vi "Drive Controller.vi"(8 "error in":errorcluster) -> ()   [LabVIEW 2015]
doc: "This VI executes continuously carrying out the current operation and responding to updates or new operation requests. It will often contain the timing or control code that is difficult to place directly in TeleOp. This VI generally opens all sensors and motors and isolates the rest of the robot code from knowing implementation details of how the operations are carried out."
uses:
  Drive Setpoints.ctl
  Drive Operations.ctl
  <vilib>/Rock Robotics/WPI/CAN/TalonSRX/WPI_CANTalonSRX_APIControlMode.ctl
  Drive Published Globals.vi
  Support Code/Team900-VIs/navX/navX Library v2/IO/Open/Z900_navX_Open_Serial.vi
  Support Code/Team900-VIs/navX/navX Library v2/navX Library v2.lvlib
  Support Code/Team900-VIs/Team900SwerveDrive/Team900SwerveDrive.lvlib
panel:
  in  "Angle Tolerances":dbl=3.0 format="%#_13g"
  in  "Ticks Per Inch":dbl=2190.379
  in  "Max Turn Speed (TPS)":dbl=2100.0
  in  "Position PID":T1
  in  "Speed PID":T1={"P"=1.0, "I"=0.004, "D"=1.296, "F Left"=0.0652246, "F Right"=0.0636451}
  in  "Max Wheel Speed (TPS)":dbl=2500.0 format="%#_13g"
  in  "Speed Setpoint (0-1)":dbl=0.4 format="%#_13g"
  out "Current Mode":dbl
  out "Position Chart":T2(graph)
  out "Speed Chart":T3(graph)
  out "Current\nCmd":string
  # "Tip: It may be helpful to observe inputs and sensor values.\nYou may also want to display tuning or debugging controls."
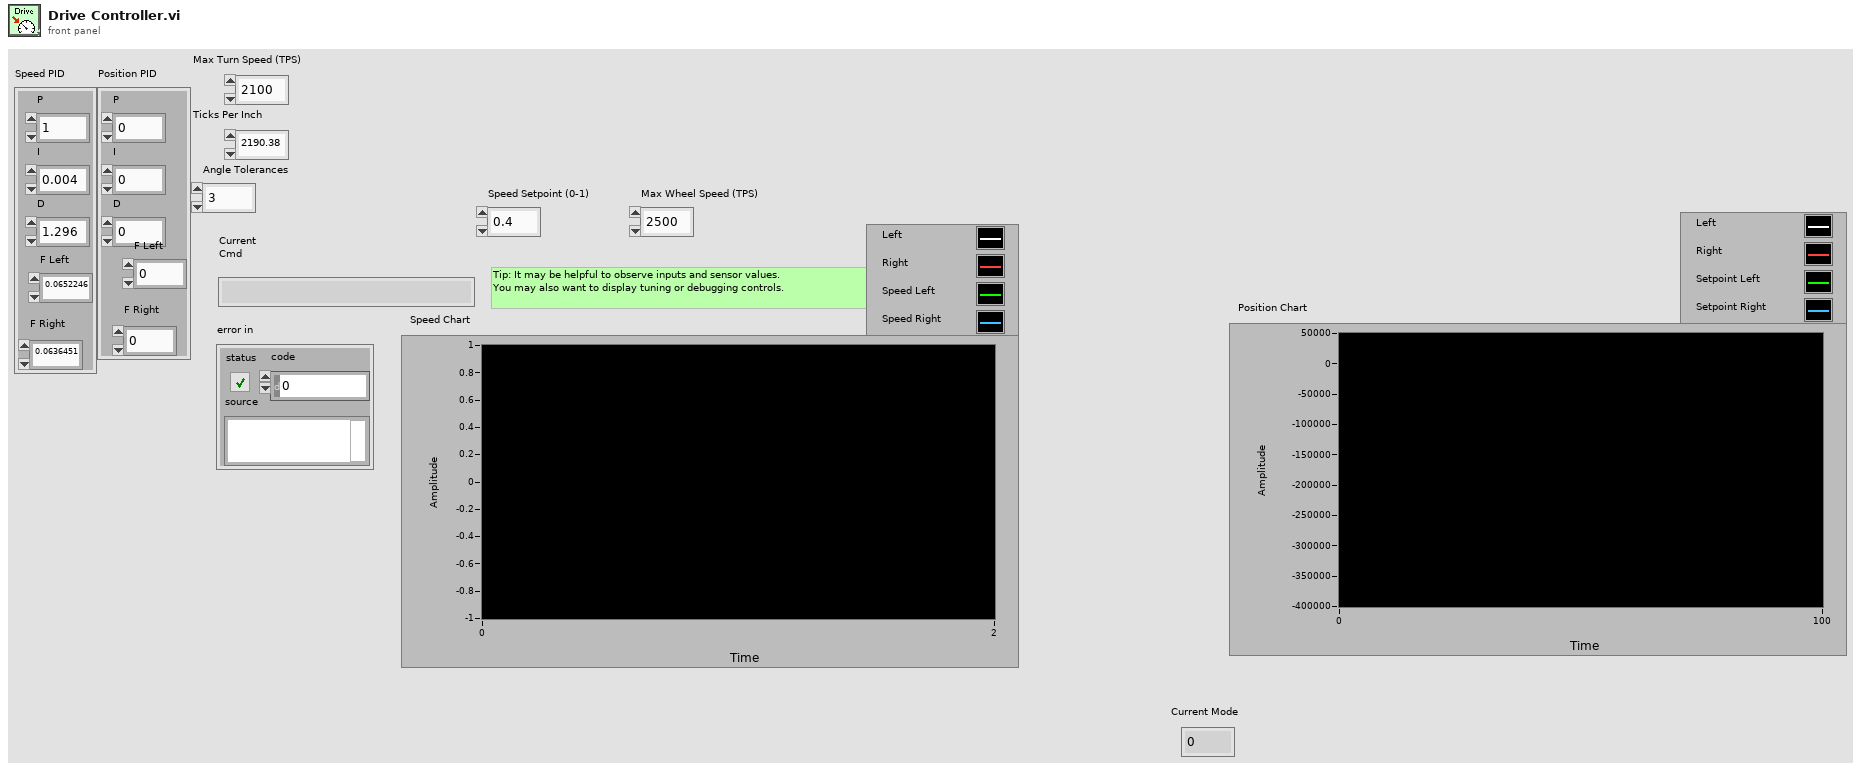
[diagram p1: front panel]
types:
  T1 = cluster{"P":dbl, "I":dbl, "D":dbl, "F Left":dbl, "F Right":dbl}
  T2 = cluster{"Sensor Velocity":dbl, "Sensor Position":dbl}
  T3 = cluster{"Sensor Velocity":dbl, "Sensor Velocity":dbl, "Sensor Velocity":dbl, "Sensor Velocity":dbl}
  T4 = typedef "Drive Setpoints.ctl" = cluster{"Operation":T5, "Left Setpoint":dbl, "Right Setpoint":dbl, "Duration":dbl, "Position":cluster{"X":dbl, "Y":dbl, "Angle":dbl}, "Face angle?":bool}
  T5 = typedef "Drive Operations.ctl" = enum16{"Reserve", "Read Current", "Immediate", "Turn Drive Turn", "Drive to Target (arc)", "Drive for Distance"}
  T6 = typedef "WPI_MotorControlDeviceRef.ctl" = cluster{"DeviceStatus":errorcluster, "Type":T7, "PWM":cluster{"PWM Channel":T8, "DeadBand":T9}, "CAN":cluster{"Device Number":u8, "Control Mode":T10, "Semaphore":T11, "Max Vout":dbl, "TalonSRX Control Mode":T12}, "Invert":bool}
  T7 = typedef "WPI_MotorControlType.ctl" = enum16{"PWM", "CAN", "CANTalonSRX"}
  T8 = typedef "FPGA_DIOPWMChannel.ctl" = enum8{"PWM 0", "PWM 1", "PWM 2", "PWM 3", "PWM 4", "PWM 5", "PWM 6", "PWM 7", "PWM 8", "PWM 9", "PWM MXP 0", "PWM MXP 1", "PWM MXP 2", "PWM MXP 3", "PWM MXP 4", "PWM MXP 5", "PWM MXP 6", "PWM MXP 7", "PWM MXP 8", "PWM MXP 9", "Invalid"}
  T9 = typedef "WPI_PWMDeadband.ctl" = cluster{"Name":string, "maxPositivePwm":i32, "minPositivePwm":i32, "centerPwm":i32, "maxNegativePwm":i32, "minNegativePwm":i32, "angularRange":u16}
  T10 = typedef "WPI_CANJaguar_ControlMode.ctl" = enum8{"Percent VBus", "Current", "Speed", "Position", "Voltage"}
  T11 = typedef "Semaphore RefNum" = refnum<k1>
  T12 = typedef "WPI_CANTalonSRX_APIControlMode.ctl" = enum8{"Percent VBus", "Speed", "Position", "Slave", "Unchanged / Invalid", "Voltage Compensation", "Current", "Motion Profile"}
  T13 = typedef "Command Status Info.ctl" = cluster{"Name":string, "Status":T14, "notifier out":T15}
  T14 = typedef "Completion Status.ctl" = enum16{"Successful", "Aborted", "Incomplete"}
  T15 = typedef "Completion Notifier.ctl" = refnum<notifier>
  T16 = cluster{"SubSystem Data":T4, cluster{"Start Time (ms)":u32, "Iterations":i32}, cluster{"Command Info":T13, "Description":string, "SubSystem Data":T4, "notifier out":refnum<notifier>, "Subsystem Name":string}}
  T17 = typedef "navX Library v2.lvlib/Z900_navX_DeviceTypeDef.ctl" = cluster{"Interface":cluster{"Protocol":T18, "Update Rate (4Hz-60Hz)":u8, "navX Open TypeDef":variant}, "Notify Packet":refnum<notifier>, "Loop VI Refnum":refnum<vi>, "Ready to Close Occurrence Refnum":refnum<k4>}
  T18 = typedef "navX Library v2.lvlib/Z900_navX_ProtocolTypeDef.ctl" = enum16{"SERIAL", "I2C", "SPI"}
  T19 = cluster{"Yaw":dbl, "Roll":dbl, "Pitch":dbl, "Heading":dbl, "Fused Heading":dbl}
  T20 = typedef "WPI_CANTalonSRX_GlobalStatus.ctl" = cluster{"Applied Throttle":dbl, "Module Enabled":bool, "CAN Error":errorcluster, "Closed Loop Error":dbl, "Forward Limit Switch Closed":bool, "Reverse Limit Switch Closed":bool, "Sensor Position":dbl, "Sensor Velocity":dbl, "Current":dbl, "Sticky Fault - Over Temp":bool, "Sticky Fault - Under Voltage":bool, "Sticky Fault - Forward Limit":bool, "Sticky Fault - Reverse Limit":bool, "Sticky Fault - Forward Soft Limit":bool, "Sticky Fault - Reverse Soft Limit":bool, "Brake is Enabled":bool, "Encoder Position":dbl, "Encoder Velocity":dbl, "Encoder Index Count":dbl, "Encoder A Pin State":bool, "Encoder B Pin State":bool, "Encoder Index Pin State":bool, "Analog In":dbl, "Analog In Velocity":dbl, "Temperature (C)":dbl, "Battery Voltage":dbl, "Control 5 Is Supported":bool, "Current Profile Slot Select":dbl, "Pos Div 8":bool, "Vel Div 4":bool, "Pulse Width Position":i32, "Pulse Width Velocity":i32, "Pulse Width Rise To Rise (us)":i32, "Pulse Width Rise To Fall (us)":i32, "Mot Prof Active Is Under Run":bool, "Mot Prof Active Has Under Run":bool, "Mot Prof Active Is Last":bool, "Mot Prof Active Velocity Only":bool, "Mot Prof Active Is Valid":bool, "Mot Prof Buffer Is Full":bool, "Mot Prof Active Profile Slot Select":i32, "Mot Prof NextID":i32, "Mot Prof Count":i32, "Mot Prof Active Velocity":dbl, "Mot Prof Active Position":dbl, "Mot Prof Output Enable":i32}
  T21 = cluster{"SubSystem Data":T4, cluster{"Start Time (ms)":u32, "Iterations":i32}, "Default Command Arguments":cluster{"Command Info":T13, "Description":string, "SubSystem Data":T4, "notifier out":refnum<notifier>, "Subsystem Name":string}}
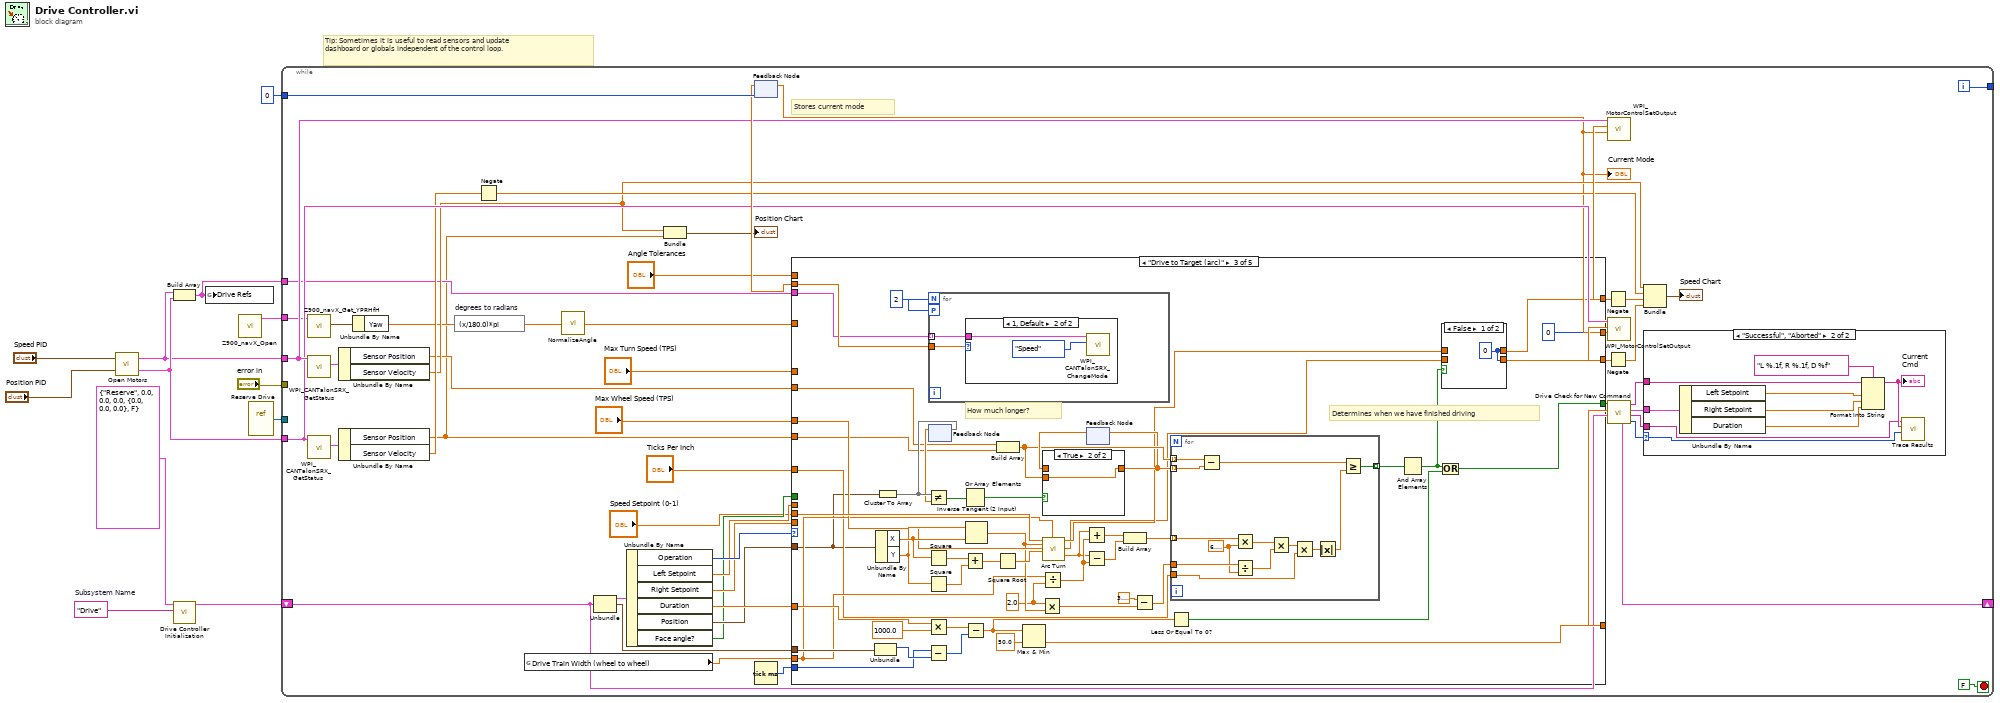
[diagram p0: block diagram]
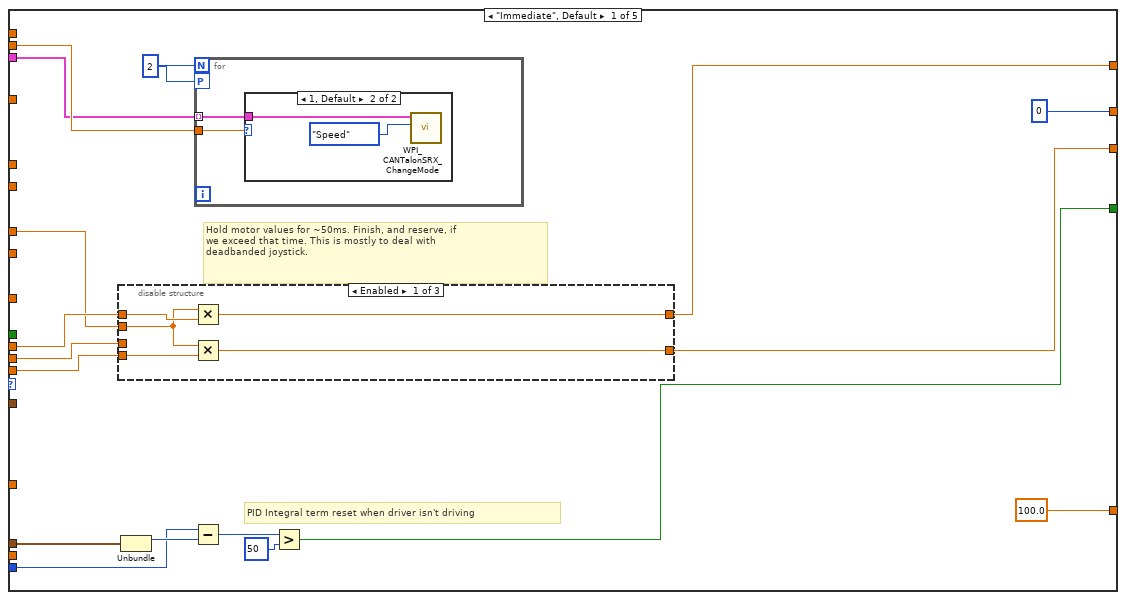
[diagram p3: hidden frame]
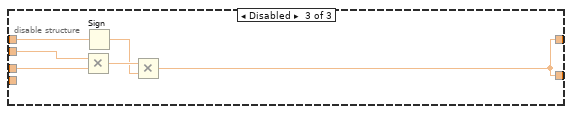
[diagram p6: hidden frame]
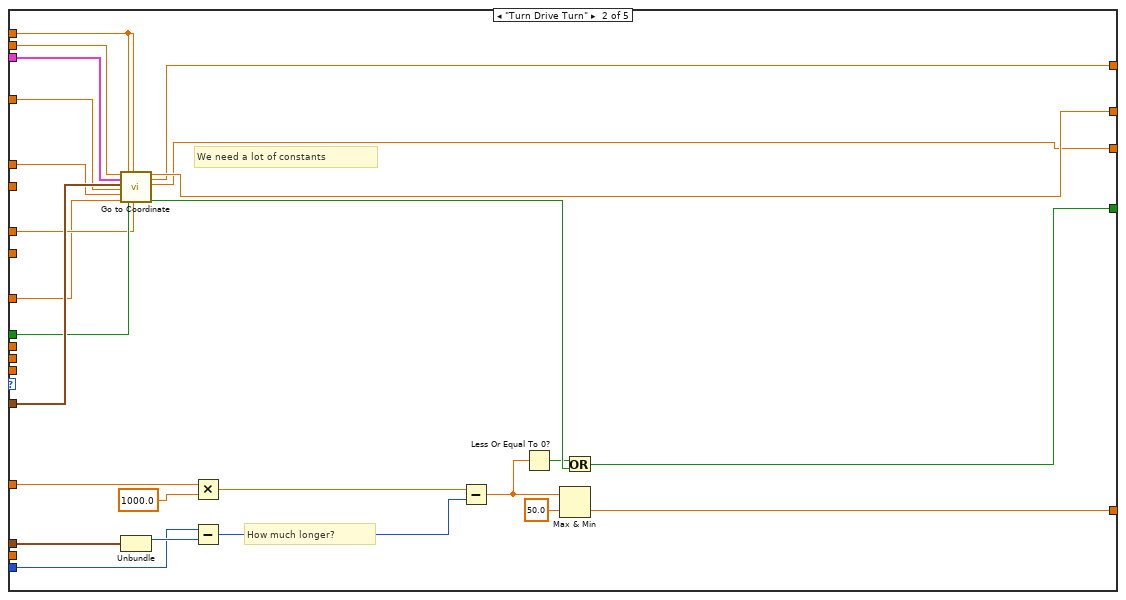
[diagram p7: hidden frame]
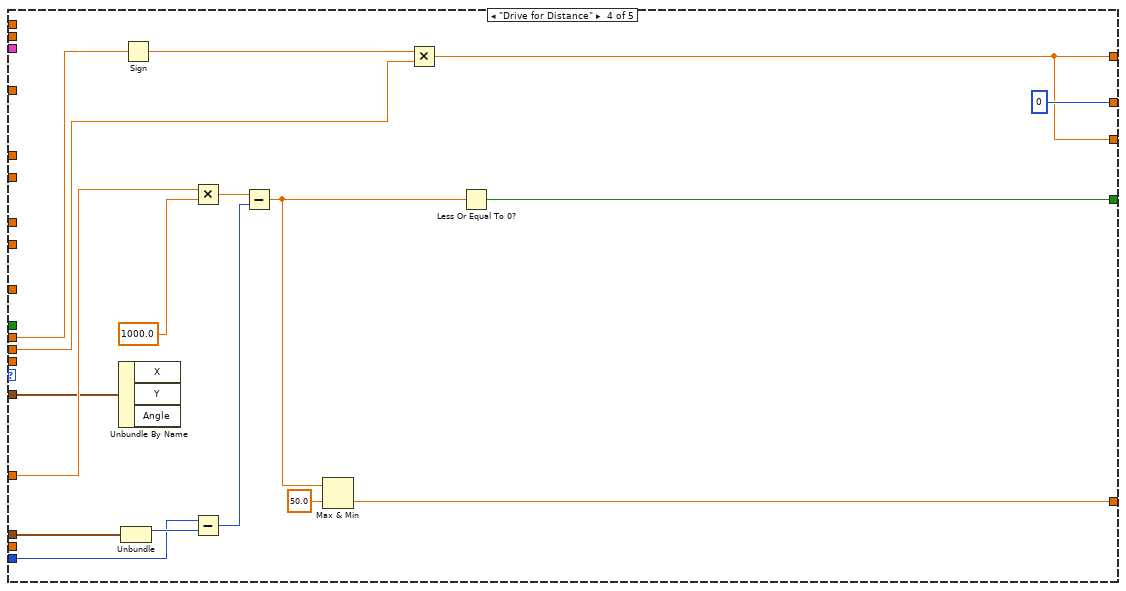
[diagram p11: hidden frame]
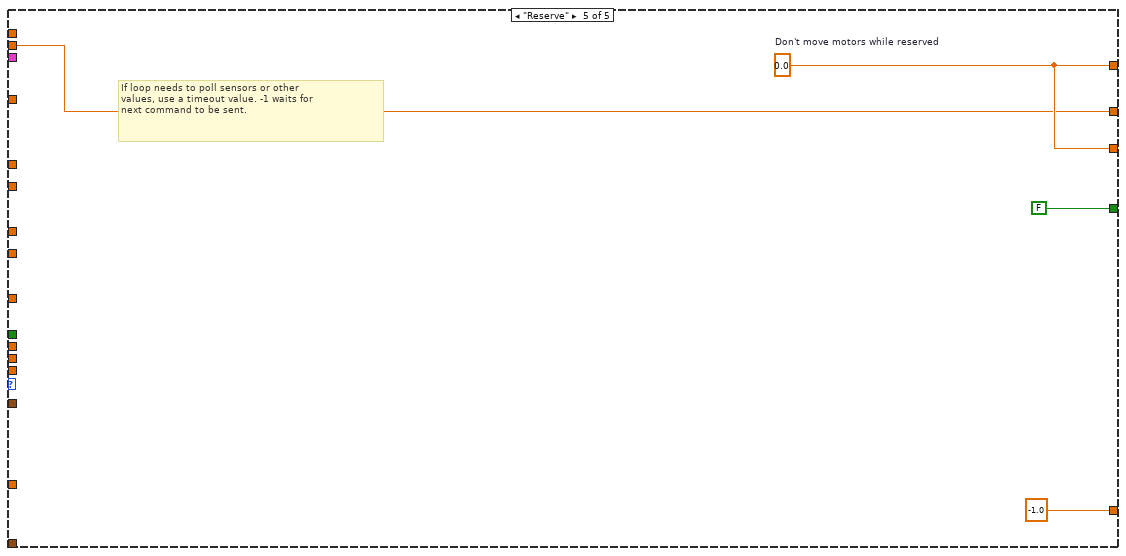
[diagram p12: hidden frame]
diagram:
  w12 = "Drive"  # Subsystem Name
  # "Tip: Sometimes it is useful to read sensors and update\ndashboard or globals independent of the control loop."
  n1 = call "Open Motors.vi"("Position PID"="Position PID", "Speed PID"="Speed PID") -> ("Right Motor Refs"=w3:T6, "Left Motor Refs"=w2:T6)
  n2 = Build Array(w2, w3) -> (w1:T6[])
  n3 = call "Drive Controller Initialization.vi"("Subsystem Name"=w12, "Default Command"=T4 {"Operation"=enum."Reserve", "Left Setpoint"=0.0, "Right Setpoint"=0.0, "Duration"=0.0, "Position"={"X"=0.0, "Y"=0.0, "Angle"=0.0}, "Face angle?"=FALSE}) -> ("output cluster"=w10:T16)  [unwired: 9 in]
  n4 = global write "Drive Published Globals.vi" "Drive Refs"(w1) -> ()
  n5 = call-poly "Z900_navX_Open.vi"() -> ("navX Device"=w7:T17)  [unwired: 10 in, 1 out]
  n6 = vi-ref "Reserve Drive.vi"() -> (w9:refnum<vi>)
  n7 = while {
    shift-right: [w52] -> _
    shift-left: w10 -> [w45]
    tunnel: [w60] -> _
    tunnel: "error in" -> [_]
    tunnel: w9 -> [_]
    tunnel: w3 -> [w36]
    tunnel: w2 -> [w37]
    tunnel: 0 -> [w43]
    tunnel: w7 -> [w25]
    tunnel: w1 -> [w19]
    i -> [w60]
    stop <- FALSE stop-if-true
    # "Stores current mode"
    n8 = call "Z900_navX_Get_YPRHfH.vi"("navX Device"=w25) -> ("YRPHfH"=w27:T19)  [unwired: 7 in, 3 out]
    n9 = call <vilib>:"WPI_CANTalonSRX_GetStatus.vi"("CAN Talon SRX Ref"=w37) -> ("Talon SRX Status"=w39:T20)  [unwired: 8 in, 2 out]
    n10 = call <vilib>:"WPI_CANTalonSRX_GetStatus.vi"("CAN Talon SRX Ref"=w36) -> ("Talon SRX Status"=w38:T20)  [unwired: 8 in, 2 out]
    n11 = Unbundle By Name(w39) -> ("Sensor Position"=w14:dbl, "Sensor Velocity"=w29:dbl)
    n12 = Unbundle By Name(w38) -> ("Sensor Position"=w13:dbl, "Sensor Velocity"=w30:dbl)
    n13 = Unbundle By Name(w27) -> ("Yaw"=w26:dbl)
    n14 = expression code="(x/180.0)*pi" "degrees to radians"(w26) -> (w24:dbl)
    n15 = Negate(x=w30) -> (-x=w34:dbl)
    n16 = global read "Drive Published Globals.vi" "Drive Train Width (wheel to wheel)"() -> (w18:dbl)
    n17 = call "NormalizeAngle.vi"("angle (rad)"=w24) -> ("angle (between pi and -pi)"=w23:dbl)
    n18 = Unbundle(w45) -> ("SubSystem Data"=w58:T4, w46:cluster{"Start Time (ms)":u32, "Iterations":i32})  [unwired: 1 out]
    n19 = Unbundle By Name(w58) -> ("Operation"=w57:T5, "Left Setpoint"=w44:dbl, "Right Setpoint"=w56:dbl, "Duration"=w55:dbl, "Position"=w41:cluster{"X":dbl, "Y":dbl, "Angle":dbl}, "Face angle?"=w40:bool)
    n20 = Bundle("Sensor Velocity"=w29, "Sensor Position"=w13) -> (→"Position Chart":T2)  [unwired: 1 in]
    n21 = feedback #1(w43) -> (w42:dbl)
    n22 = Tick Count (ms)() -> (millisecond timer value=w54:u32)
    n23 = case shown="\"Drive to Target (arc)\"" w57 {
      tunnel: [100.0 w120 w166 w210 -1.0] -> w51
      tunnel: [w82 w113 w136 w211 FALSE ("ignore previous (F)")] -> w50
      tunnel: w46 -> [w81 w126 w171 w213 _]
      tunnel: [w72 w111 w135 w204 w222] -> w35
      tunnel: [w73 w110 w133 w204 w222] -> w33
      tunnel: w56 -> [w80 _ _ _ _]
      tunnel: w55 -> [_ w124 w169 w214 _]
      tunnel: w54 -> [w83 w123 w172 w212 _]
      tunnel: w44 -> [w79 _ _ w208 _]
      tunnel: [0 w118 0 0 w221] -> w20
      tunnel: w42 -> [w78 w117 w164 _ w221]
      tunnel: w19 -> [w77 w119 w163 _ _]
      tunnel: w41 -> [_ w116 w148 w209 _]
      tunnel: w40 -> [_ w115 _ _ _]
      tunnel: w23 -> [_ w109 _ _ _]
      tunnel: "Speed Setpoint (0-1)" -> [w74 _ w161 w205 _]
      tunnel: "Max Wheel Speed (TPS)" -> [w76 w108 w160 _ _]
      tunnel: w18 -> [_ _ w154 _ _]
      tunnel: "Max Turn Speed (TPS)" -> [_ w107 _ _ _]
      tunnel: "Ticks Per Inch" -> [_ w106 w153 _ _]
      tunnel: "Angle Tolerances" -> [_ w105 _ _ _]
      tunnel: w14 -> [_ _ w143 _ _]
      tunnel: w13 -> [_ _ w142 _ _]
      frame "Immediate", Default {
        w71 = 2
        # "PID Integral term reset when driver isn't driving"
        # "Hold motor values for ~50ms. Finish, and reserve, if\nwe exceed that time. This is mostly to deal with\ndeadbanded joystick."
        n24 = disable-structure shown="Enabled" {
          disable-tunnel: w80 -> [w96 w97 _]
          disable-tunnel: [w95 w97 w101] -> w73
          disable-tunnel: w79 -> [w94 w98 w100]
          disable-tunnel: [w93 w98 w101] -> w72
          disable-tunnel: w76 -> [w92 _ w104]
          disable-tunnel: w74 -> [_ _ w103]
          frame Enabled {
            n25 = Multiply(x=w92, y=w94) -> (x*y=w93:dbl)
            n26 = Multiply(x=w92, y=w96) -> (x*y=w95:dbl)
          }
          frame Disabled {
          }
          frame Disabled {
            n27 = Multiply(x=w104, y=w103) -> (x*y=w102:dbl)
            n28 = Sign(1:w100) -> (0:w99:dbl)
            n29 = Multiply(x=w102, y=w99) -> (x*y=w101:dbl)
          }
        }
        n30 = Unbundle(w81) -> ("Start Time (ms)"=w84:u32)  [unwired: 1 out]
        n31 = Subtract(x=w83, y=w84) -> (x-y=w85:u32)
        n32 = for {
          N: w71 -> [_]
          tunnel: w78 -> [w89]
          tunnel: w77 -> [w88] mode=indexing
          workers-P: w71 -> [_]
          n33 = case shown="1, Default" w89 {
            tunnel: w88 -> [_ w91]
            frame 0 {
            }
            frame 1, Default {
              n34 = call <vilib>:"WPI_CANTalonSRX_ChangeMode.vi"("Control Mode"=WPI_CANTalonSRX_APIControlMode."Speed", "CAN Talon SRX Ref"=w91) -> ()  [unwired: 8 in, 2 out]
            }
          }
        }
        n35 = Greater?(x=w85, y=u8 50 ("Left Motor")) -> (0:w82:bool)
      }
      frame "Turn Drive Turn" {
        # "We need a lot of constants"
        # "How much longer?"
        n36 = call "Go to Coordinate.vi"("Current Mode"=w117, "Motor Refs"=w119, "Position"=w116, "Current Angle (radians; 0 = right)"=w109, "Max Turn Speed (TPS)"=w107, "Ticks Per Inch"=w106, "Angle Tolerances 1"=w105, "Face angle?"=w115, "Angle Tolerances 2"=w105, "Max  Wheel Speed (TPS)"=w108) -> ("New Mode"=w118:dbl, "Left Setpoint"=w111:dbl, "Right Setpoint"=w110:dbl, "Finished?"=w114:bool)  [unwired: 6 in]
        n37 = Unbundle(w126) -> ("Start Time (ms)"=w125:u32)  [unwired: 1 out]
        n38 = Multiply(x=w124, y=1000.0) -> (x*y=w128:dbl)
        n39 = Subtract(x=w123, y=w125) -> (x-y=w129:u32)
        n40 = Subtract(x=w128, y=w129) -> (x-y=w122:dbl)
        n41 = Less Or Equal To 0?(x=w122) -> (x <= 0?=w112:bool)
        n42 = Max & Min(x=w122, y=50.0) -> (min(x,y)=w120:dbl)  [unwired: 1 out]
        n43 = Or(x=w112, y=w114) -> (x .or. y?=w113:bool)
      }
      frame "Drive to Target (arc)" {
        w155 = 2.0 ("x")
        w165 = 2
        # "Determines when we have finished driving"
        # "How much longer?"
        n44 = Unbundle(w171) -> ("Start Time (ms)"=w174:u32)  [unwired: 1 out]
        n45 = Unbundle By Name(w148) -> ("X"=w181:dbl, "Y"=w180:dbl)
        n46 = Cluster To Array(cluster=w148) -> (array=w147:dbl[])
        n47 = Square(x=w181) -> (x^2=w177:dbl)
        n48 = Square(x=w180) -> (x^2=w179:dbl)
        n49 = Multiply(x=w169, y=1000.0) -> (x*y=w168:dbl)
        n50 = Subtract(x=w172, y=w174) -> (x-y=w175:u32)
        n51 = for {
          N: w165 -> [_]
          tunnel: w164 -> [w201]
          tunnel: w163 -> [w200] mode=indexing
          workers-P: w165 -> [_]
          n52 = case shown="1, Default" w201 {
            tunnel: w200 -> [_ w203]
            frame 0 {
            }
            frame 1, Default {
              n53 = call <vilib>:"WPI_CANTalonSRX_ChangeMode.vi"("Control Mode"=WPI_CANTalonSRX_APIControlMode."Speed", "CAN Talon SRX Ref"=w203) -> ()  [unwired: 8 in, 2 out]
            }
          }
        }
        n54 = feedback-in #2(w147) -> ()
        n55 = feedback #2() -> (w146:dbl[])  [unwired: 1 in]
        n56 = Not Equal?(x=w147, y=w146) -> (x != y?=w145:bool[])
        n57 = Or Array Elements(Boolean array=w145) -> (logical OR=w144:bool)
        n58 = Add(x=w177, y=w179) -> (x+y=w178:dbl)
        n59 = Subtract(x=w168, y=w175) -> (x-y=w167:dbl)
        n60 = Inverse Tangent (2 Input)(1:w181, 2:w180) -> (0:w157:dbl)
        n61 = Square Root(x=w178) -> (sqrt(x)=w176:dbl)
        n62 = Build Array(w143, w142) -> (w140:dbl[])
        n63 = Max & Min(x=w167, y=50.0) -> (min(x,y)=w166:dbl)  [unwired: 1 out]
        n64 = Multiply(x=w155, y=w157) -> (x*y=w158:dbl)
        n65 = Divide(x=w154, y=w155) -> (x/y=w152:dbl)
        n66 = call "Arc Turn.vi"("Speed Setpoint (0-1)"=w161, "Angle Radians (0 = Right)"=w157, "Max Speed (TPS)"=w160, "Distance"=w176, "Robot Width"=w154) -> ("Left Speed"=w134:dbl, "Right Speed"=w132:dbl, "Radius"=w130:dbl)  [unwired: 12 in]
        n67 = Add(x=w130, y=w152) -> (x+y=w151:dbl)
        n68 = Subtract(x=w130, y=w152) -> (x-y=w150:dbl)
        n69 = feedback #3() -> (w141:dbl[])  [unwired: 1 in]
        n70 = case shown="True" w144 {
          tunnel: [w185 w186] -> w139
          tunnel: w140 -> [_ w186]
          tunnel: w141 -> [w185 _]
          frame False {
          }
          frame True {
          }
        }
        n71 = feedback-in #3(w139) -> ()
        n72 = Build Array(w151, w150) -> (w149:dbl[])
        n73 = Subtract(x=3.141592653589793, y=w158) -> (x-y=w156:dbl)
        n74 = Less Or Equal To 0?(x=w167) -> (x <= 0?=w137:bool)
        n75 = for {
          tunnel: w156 -> [w199]
          tunnel: w153 -> [w196]
          tunnel: w149 -> [w193] mode=indexing
          tunnel: w140 -> [w192] mode=indexing
          tunnel: w139 -> [w191] mode=indexing
          tunnel: [w189] -> w138 mode=indexing
          w197 = 6.283185307179586
          n76 = Subtract(x=w192, y=w191) -> (x-y=w190:dbl)
          n77 = Multiply(x=w193, y=w197) -> (x*y=w195:dbl)
          n78 = Divide(x=w199, y=w197) -> (x/y=w198:dbl)
          n79 = Multiply(x=w195, y=w198) -> (x*y=w194:dbl)
          n80 = Multiply(x=w194, y=w196) -> (x*y=w188:dbl)
          n81 = Absolute Value(x=w188) -> (abs(x)=w187:dbl)
          n82 = Greater Or Equal?(x=w190, y=w187) -> (x >= y?=w189:bool)
        }
        n83 = And Array Elements(Boolean array=w138) -> (logical AND=w131:bool)
        n84 = Or(x=w131, y=w137) -> (x .or. y?=w136:bool)
        n85 = case shown="False" w131 {
          tunnel: [w182 w184] -> w135
          tunnel: w134 -> [_ w184]
          tunnel: [w182 w183] -> w133
          tunnel: w132 -> [_ w183]
          frame False {
            w182 = 0
          }
          frame True {
          }
        }
      }
      frame "Drive for Distance" {
        n86 = Unbundle By Name(w209) -> ()  [unwired: 3 out]
        n87 = Unbundle(w213) -> ("Start Time (ms)"=w219:u32)  [unwired: 1 out]
        n88 = Sign(1:w208) -> (0:w207:dbl)
        n89 = Multiply(x=w214, y=1000.0) -> (x*y=w216:dbl)
        n90 = Subtract(x=w212, y=w219) -> (x-y=w220:u32)
        n91 = Subtract(x=w216, y=w220) -> (x-y=w215:dbl)
        n92 = Max & Min(x=w215, y=50.0) -> (min(x,y)=w210:dbl)  [unwired: 1 out]
        n93 = Multiply(x=w207, y=w205) -> (x*y=w204:dbl)
        n94 = Less Or Equal To 0?(x=w215) -> (x <= 0?=w211:bool)
      }
      frame "Reserve" {
        w222 = 0.0  # Don't move motors while reserved
        # "If loop needs to poll sensors or other\nvalues, use a timeout value. -1 waits for\nnext command to be sent."
      }
    }
    "Current Mode" <- w20
    n95 = feedback-in #1(w20) -> ()
    n96 = Negate(x=w35) -> (-x=w32:dbl)
    n97 = Negate(x=w33) -> (-x=w31:dbl)
    n98 = call <vilib>:"WPI_MotorControlSetOutput.vi"("Sync Group / Parameter Slot"=w20, "Output"=w35, "MotorControlDevRef"=w37) -> ()  [unwired: 6 in, 3 out]
    n99 = call <vilib>:"WPI_MotorControlSetOutput.vi"("Sync Group / Parameter Slot"=w20, "Output"=w33, "MotorControlDevRef"=w36) -> ()  [unwired: 6 in, 3 out]
    n100 = call "Drive Check for New Command.vi"("input cluster"=w45, "Wait time (ms)"=w51, "Finished?"=w50) -> ("Completion"=w53:T14, "Subsystem Name"=w47:string, "SetPoint"=w48:T4, "Initial Trace String"=w49:string, "output cluster"=w52:T21)  [unwired: 4 in]
    n101 = Bundle("Sensor Velocity"=w29, w34, w32, w31) -> (→"Speed Chart":cluster{"Sensor Velocity":dbl, dbl, dbl, dbl})  [unwired: 1 in]
    n102 = case shown="\"Successful\", \"Aborted\"" w53 {
      selector: w53 -> [_ w70]
      tunnel: w49 -> [_ w65]
      tunnel: w48 -> [_ w66]
      tunnel: w47 -> [_ w62]
      frame "Incomplete", Default {
        # "Continuing current command"
      }
      frame "Successful", "Aborted" {
        # "Report and setup for next command"
        n103 = Unbundle By Name(w66) -> ("Left Setpoint"=w68:dbl, "Right Setpoint"=w69:dbl, "Duration"=w63:dbl)
        n104 = Format Into String(format string="L %.1f, R %.1f, D %f", initial string=w65, w68, w69, w63) -> (resulting string=w64:string)  [unwired: 1 in, 1 out]
        "Current\nCmd" <- w64
        n105 = call <vilib>:"Trace Results.vi"("Status of previous command"=w70, "Description"=w64, "Subsystem"=w62) -> ()  [unwired: 9 in]
      }
    }
  }
